vi "TargetNTHandshake.vi"(8 "error in":errorcluster, 10 "Timeout":i32=10000, 11 "Name":string="Boolean") -> (0 "error out":errorcluster, 3 "Acknowledged":bool)   [LabVIEW 2016]
uses:
  <vilib>/Rock Robotics/Network Tables/NT Write Boolean.vi
  <vilib>/Rock Robotics/Network Tables/NT Read Boolean.vi
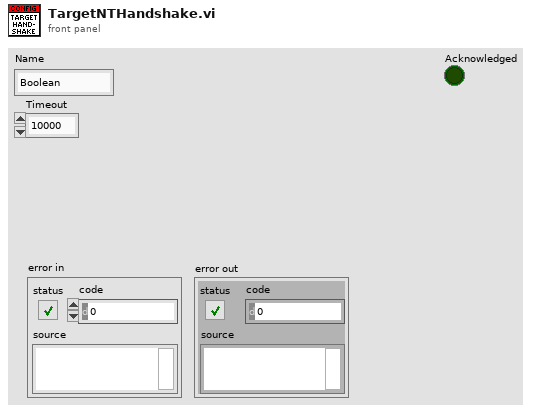
[diagram p1: front panel]
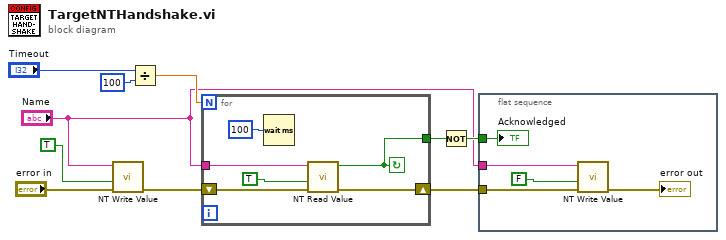
[diagram p0: block diagram]
diagram:
  n1 = call-poly <vilib>:"NT Write Value.vi"("error in"="error in", "Boolean"=TRUE, "Name"="Name") -> ("error out"=w6:errorcluster)  [unwired: 8 in]
  n2 = Divide(x="Timeout", y=100) -> (x/y=w9:dbl)
  n3 = for {
    N: w9 -> [_]
    tunnel: "Name" -> [w14]
    tunnel: [w12] -> w4
    shift-right: [w11] -> w2
    shift-left: w6 -> [w15]
    stop <- w12 continue-if-true
    n4 = Wait (ms)(milliseconds to wait=u32 100) -> ()  [unwired: 1 out]
    n5 = call-poly <vilib>:"NT Read Value.vi"("error in"=w15, "Default Value"=TRUE, "Name"=w14) -> ("error out"=w11:errorcluster, "Boolean"=w12:bool)  [unwired: 7 in]
  }
  n6 = Not(x=w4) -> (.not. x?=w3:bool)
  n7 = flat-sequence {
    tunnel: w3 -> [w21]
    tunnel: w2 -> [w19]
    tunnel: "Name" -> [w17]
    frame #0 {
      n8 = call-poly <vilib>:"NT Write Value.vi"("error in"=w19, "Boolean"=FALSE, "Name"=w17) -> ("error out"=→"error out":errorcluster)  [unwired: 8 in]
      "Acknowledged" <- w21
    }
  }
